vi "Make AO JSON.vi"(9 "Force":bool, 10 "AO prev":T1={"type"="AO", "device"="", "name"="", "data"={"<init"=FALSE, "<voltage"=0.0}}, 11 "AO new":T1={"type"="AO", "device"="", "name"="", "data"={"<init"=FALSE, "<voltage"=0.0}}) -> (3 "delta JSON":string)   [LabVIEW 2019]
uses:
  AO proto.ctl
  AO Data proto.ctl
panel:
  out "Complete JSON":string
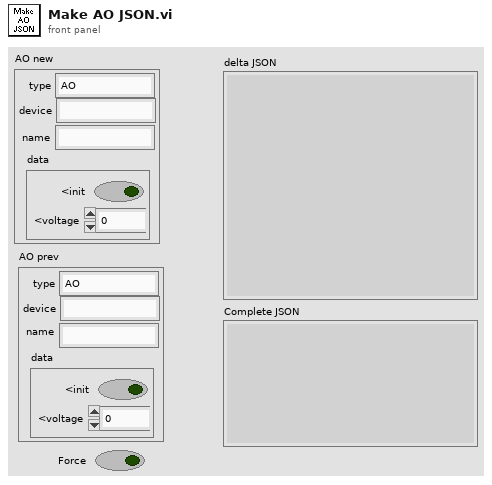
[diagram p1: front panel]
types:
  T1 = typedef "AO proto.ctl" = cluster{"type":string, "device":string, "name":string, "data":T2}
  T2 = typedef "AO Data proto.ctl" = cluster{"<init":bool, "<voltage":dbl}
  T3 = cluster{"type":bool, "device":bool, "name":bool, "data":cluster{"<init":bool, "<voltage":bool}}
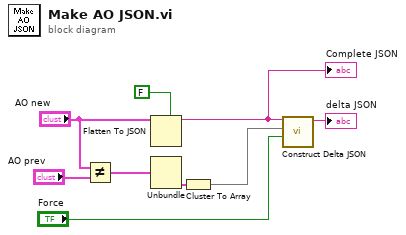
[diagram p0: block diagram]
diagram:
  n1 = Not Equal?(x="AO new", y="AO prev") -> (x != y?=w5:T3)
  n2 = Flatten To JSON(enable LabVIEW extensions? (T)=FALSE, anything="AO new") -> (JSON string=w4:string)  [unwired: 1 in, 1 out]
  "Complete JSON" <- w4
  n3 = Unbundle(w5) -> ("data"=w6:cluster{"<init":bool, "<voltage":bool})  [unwired: 3 out]
  n4 = Cluster To Array(cluster=w6) -> (array=w3:bool[])
  n5 = call "Construct Delta JSON.vi"("Force"="Force", "Checked Items"=w3, "JSON string"=w4) -> ("Delta JSON"=→"delta JSON":string)  [unwired: 8 in]
